vi "verify.vi"(0 "HGF_GPG":refnum<class "HGF_GPG.lvclass">, 1 "options file":path, 2 "keyringfile":path, 3 "Sec keyringfile":path, 4 "string in":string, 5 "error in (no error)":errorcluster, 6 "Trust DB":path) -> (8 "dup Trust DB":path, 10 "trusted":bool, 11 "success":bool=TRUE, 12 "Key-ID":string, 13 "data error":bool, 14 "dup HGF_GPG":refnum<class "HGF_GPG.lvclass">, 15 "dup options file":path, 16 "dup keyringfile":path, 17 "dup Sec keyringfile":path, 18 "String":string, 19 "error out":errorcluster)   [LabVIEW 2012, in "HGF_GPG.lvlib" / "HGF_GPG.lvclass"]
doc: "Verify A String.\nString will be encrypted. If the signature is made by a trusted key, trusted is set to true."
uses:
  HGF_GPG.lvclass
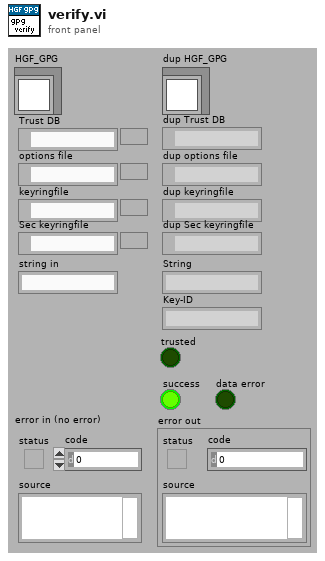
[diagram p1: front panel]
types:
  T1 = enum16{"open", "replace", "create", "open or create", "replace or create", "replace or create with confirmation"}
  T2 = enum16{"encrypt", "decrypt", "sign", "verify", "sign & encrypt", "verify & decrypt"}
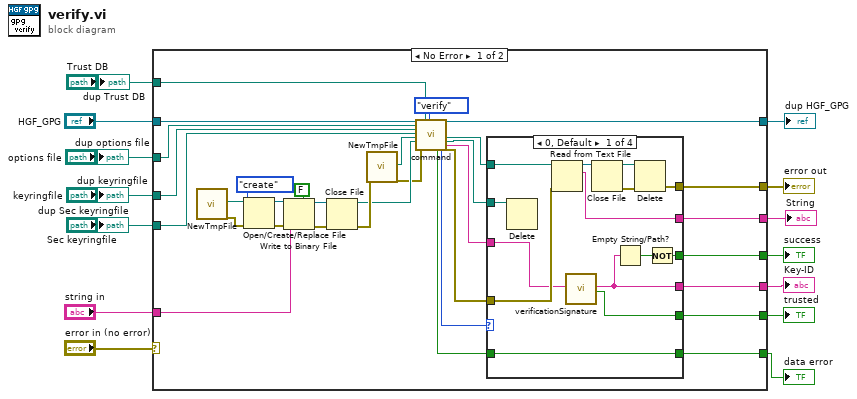
[diagram p0: block diagram]
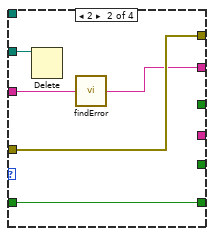
[diagram p2: hidden frame]
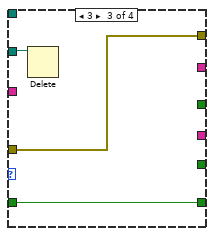
[diagram p3: hidden frame]
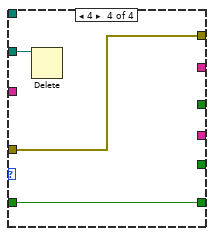
[diagram p4: hidden frame]
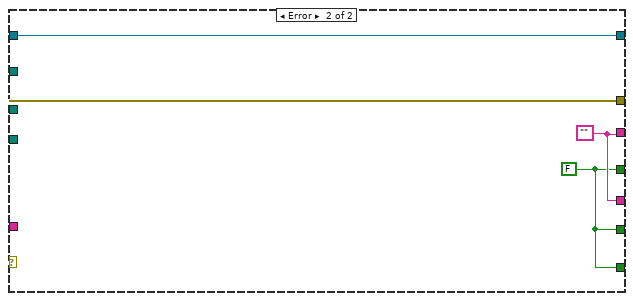
[diagram p5: hidden frame]
diagram:
  n1 = case shown="No Error" "error in (no error)" {
    selector: "error in (no error)" -> [_ w73]
    tunnel: [w44 w74] -> w12
    tunnel: "HGF_GPG" -> [w45 w74]
    tunnel: "string in" -> [w33 _]
    tunnel: [w38 w75] -> w10
    tunnel: [w37 w73] -> w9
    tunnel: [w34 w72] -> w8
    tunnel: [w32 w75] -> w7
    tunnel: [w31 w72] -> w6
    tunnel: "options file" -> [w28 _]
    tunnel: "keyringfile" -> [w27 _]
    tunnel: [w23 w72] -> w3
    tunnel: "Sec keyringfile" -> [w22 _]
    tunnel: "Trust DB" -> [w15 _]
    frame No Error {
      n2 = call "NewTmpFile.vi"() -> ("path"=w20:path, "error out"=w19:errorcluster)  [unwired: 1 in, 17 out]
      n3 = Open/Create/Replace File(file path (use dialog)=w20, error in=w19, operation (0:open)=T1."create") -> (refnum out=w16:refnum<file>, error out=w17:errorcluster)  [unwired: 4 out]
      n4 = Write to Binary File(file (use dialog)=w16, data=w33, error in=w17, 5:FALSE ("prepend array or string size? (T)")) -> (refnum out=w42:refnum<file>, error out=w43:errorcluster)  [unwired: 3 out]
      n5 = Close File(refnum=w42, error in=w43) -> (path=w29:path, error out=w46:errorcluster)
      n6 = call "NewTmpFile.vi"("error in (no error)"=w46) -> ("path"=w21:path, "error out"=w18:errorcluster)  [unwired: 17 out]
      n7 = call-dynamic "command.vi"("HGF_GPG"=w45, "options file"=w28, "keyringfile"=w27, "Sec keyringfile"=w22, "targetfile"=w21, "sourcefile"=w29, "error in (no error)"=w18, "Trust DB"=w15, "task"=T2."verify") -> ("data error"=w39:bool, "return code"=w25:i32, "dup HGF_GPG"=w44:refnum<class "HGF_GPG.lvclass">, "dup targetfile"=w26:path, "dup sourcefile"=w24:path, "standard error"=w41:string, "error out"=w40:errorcluster)  [unwired: 4 in, 8 out]
      n8 = case shown="0, Default" w25 {
        tunnel: w41 -> [w54 w63 _ _]
        tunnel: w40 -> [w56 w65 w68 w71]
        tunnel: w39 -> [w55 w64 w67 w70]
        tunnel: [w50 w62 _ _] -> w38
        tunnel: [w57 w65 w68 w71] -> w37
        tunnel: [w55 w64 w67 w70] -> w34
        tunnel: [w47 _ _ _] -> w32
        tunnel: [w53 _ _ _] -> w31
        tunnel: w26 -> [w52 _ _ _]
        tunnel: w24 -> [w51 w61 w66 w69]
        tunnel: [w48 _ _ _] -> w23
        frame 0, Default {
          n9 = Delete(path (use dialog)=w51) -> ()  [unwired: 1 in, 6 out]
          n10 = Read from Text File(file (use dialog)=w52, error in=w56) -> (refnum out=w60:refnum<file>, text=w50:string)  [unwired: 4 out]
          n11 = call "verificationSignature.vi"("String"=w54) -> ("Key-ID"=w47:string, "trusted"=w53:bool)  [unwired: 17 out]
          n12 = Close File(refnum=w60) -> (path=w58:path, error out=w59:errorcluster)  [unwired: 1 in]
          n13 = Empty String/Path?(string/path=w47) -> (empty?=w49:bool)
          n14 = Delete(path (use dialog)=w58, error in=w59) -> (error out=w57:errorcluster)  [unwired: 5 out]
          n15 = Not(x=w49) -> (.not. x?=w48:bool)
        }
        frame 2 {
          n16 = Delete(path (use dialog)=w61) -> ()  [unwired: 1 in, 6 out]
          n17 = call "findError.vi"("error string in"=w63) -> ("error out"=w62:string)
        }
        frame 3 {
          n18 = Delete(path (use dialog)=w66) -> ()  [unwired: 1 in, 6 out]
        }
        frame 4 {
          n19 = Delete(path (use dialog)=w69) -> ()  [unwired: 1 in, 6 out]
        }
      }
    }
    frame Error {
      w72 = FALSE
      w75 = ""
    }
  }
  "dup HGF_GPG" <- w12
  "String" <- w10
  "error out" <- w9
  "success" <- w3
  "data error" <- w8
  "Key-ID" <- w7
  "trusted" <- w6
  "dup options file" <- "options file"
  "dup keyringfile" <- "keyringfile"
  "dup Sec keyringfile" <- "Sec keyringfile"
  "dup Trust DB" <- "Trust DB"
